vi "Acquire.vi"(8 "error in (no error)":errorcluster, 11 "Standard Measurement in":refnum<class "Standard Measurement.lvclass">) -> (0 "error out":errorcluster, 3 "Standard Measurement out":refnum<class "Standard Measurement.lvclass">)   [LabVIEW 2026, in "Standard Measurement Plugin.lvlib" / "Standard Measurement.lvclass"]
uses:
  Standard Measurement.lvclass
  MAL-Framework/user.lib/Common Components/Measurement Actor/Measurement.lvclass
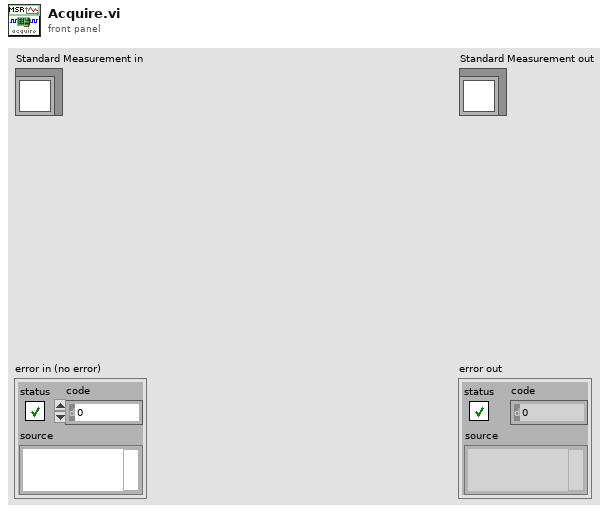
[diagram p1: front panel]
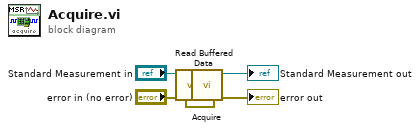
[diagram p0: block diagram]
diagram:
  n1 = call "Read Buffered Data.vi"("error in (no error)"="error in (no error)", "Standard Measurement in"="Standard Measurement in") -> ("error out"=w1:errorcluster, "Standard Measurement out"=w3:refnum<class "Standard Measurement.lvclass">)  [unwired: 8 in]
  n2 = call-parent "Acquire.vi"("error in (no error)"=w1, "Measurement in"=w3) -> ("error out"=→"error out":errorcluster, "Measurement out"=→"Standard Measurement out":refnum<class "Standard Measurement.lvclass">)  [unwired: 8 in]
